vi "FRC Retroreflective Processing Example.vi"(10 "Image Src":T2) -> ()   [LabVIEW 2014]
uses:
  Vision Support Code/Camera Types.ctl
  <vilib>/vision/Image Controls.llb/IMAQ Image.ctl
  <vilib>/vision/NI_Vision_Development_Module.lvlib
panel:
  out "Found Totes":T1(array[cluster])
  in  "Camera Type":T3=enum."MS HD3000 square"
  in  "Aspect Fudge Factor":dbl=1.0
  in  "Score Threshold":dbl=75.0
  in  "Annotate":bool=TRUE
  out "ms to process":u32
  out "Sorted Scores":T4(array[cluster]) {"Aspect Ratio" format="%#_3g"; "Area Score" format="%#_3g"; "X" format="%#_3g"; "Y" format="%#_3g"}
  out "Particles":i32
  in  "Ring Light Color":T5={"Hue"={101.37467765958063, 64.10933859299683}, "Sat"={88.03571428571429, 255.0}, "Val"={133.57142857142858, 255.0}} {"Hue" scale=0.0..255.0 scale format="%#_3g"}
  out "Masked":T2(plugin-control)
  out "Original Image":T2(plugin-control)
  # "Instructions:\nUse Source to select image files from a directory or use a USB or IP camera connected to your laptop.\nUse the Color of a ring light to threshold and build particles. Adjust calibration if needed.\nSmall modifications to the diagram will allow for intensity processing instead of color.\nAnnotations show the rectangle and the scores from top to bottom."
  # "Density Profile"
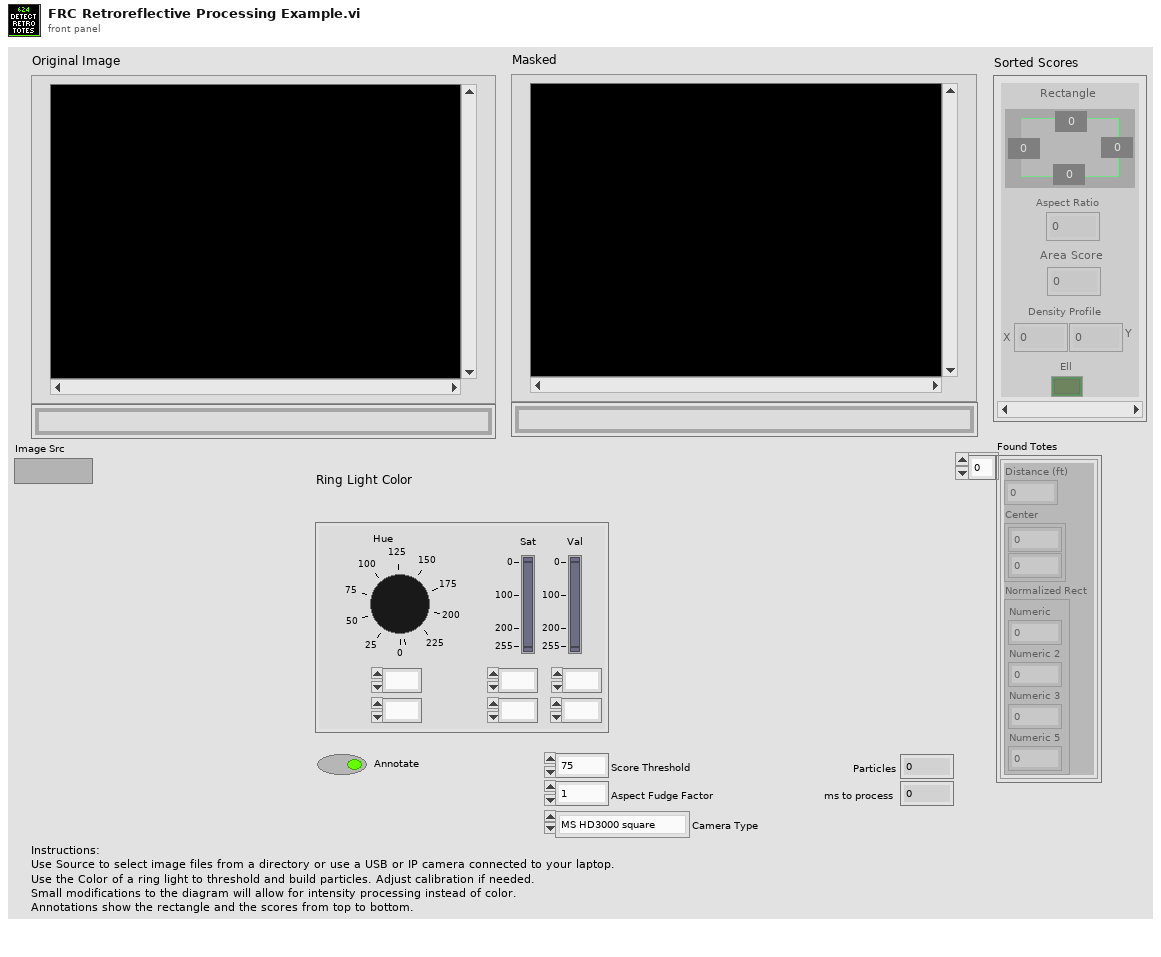
[diagram p1: front panel]
types:
  T1 = cluster{"Distance (ft)":dbl, "Center":cluster{dbl, dbl}, "Normalized Rect":cluster{"Numeric":dbl, "Numeric 2":dbl, "Numeric 3":dbl, "Numeric 5":dbl}}[]
  T2 = typedef "IMAQ Image.ctl" = refnum<image>
  T3 = typedef "Camera Types.ctl" = enum16{"206", "1011", "1013", "MS HD3000 square", "MS HD3000 640x480"}
  T4 = cluster{"Rectangle":cluster{"Numeric":dbl, "Numeric 2":dbl, "Numeric 3":dbl, "Numeric 5":dbl}, "Aspect Ratio":dbl, "Area Score":dbl, "X":dbl, "Y":dbl, "Ell":bool}[]
  T5 = cluster{"Hue":cluster{dbl, dbl}, "Sat":cluster{dbl, dbl}, "Val":cluster{dbl, dbl}}
  T6 = typedef "Particle Parameters" = i32
  T7 = typedef "Image Type" = u32
  T8 = cluster{"Bounding box":cluster{"left":dbl, "top":dbl, "right":dbl, "bottom":dbl}, "Aspect Ratio":dbl, "Area Score":dbl, "X Mask":dbl, "Y Mask":dbl, "Ell":bool}[]
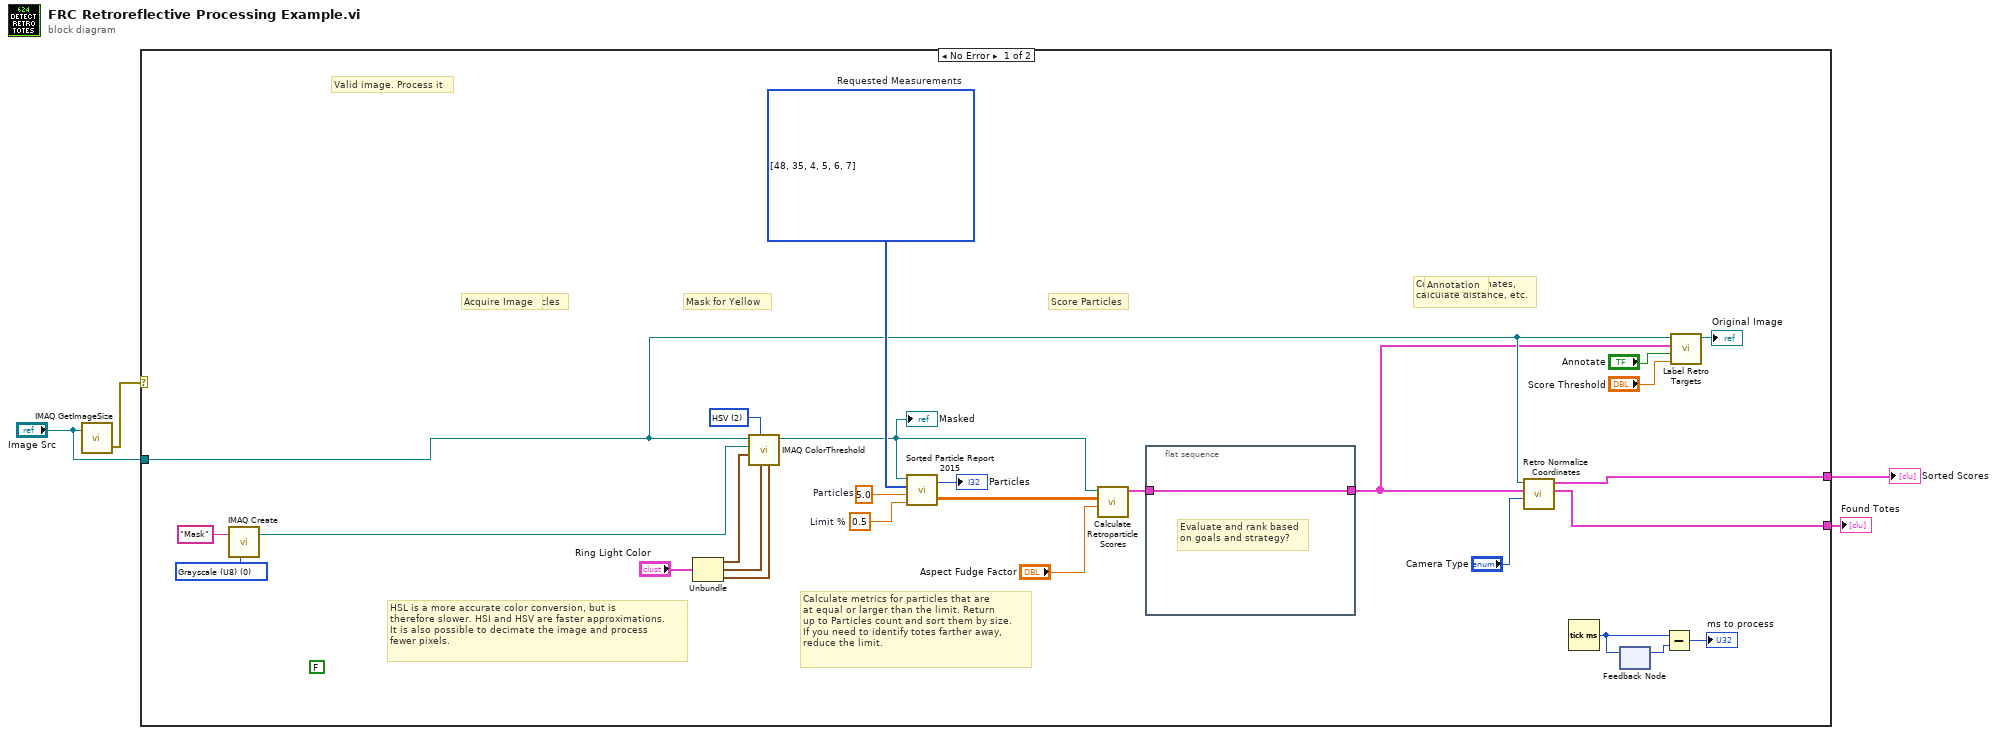
[diagram p0: block diagram]
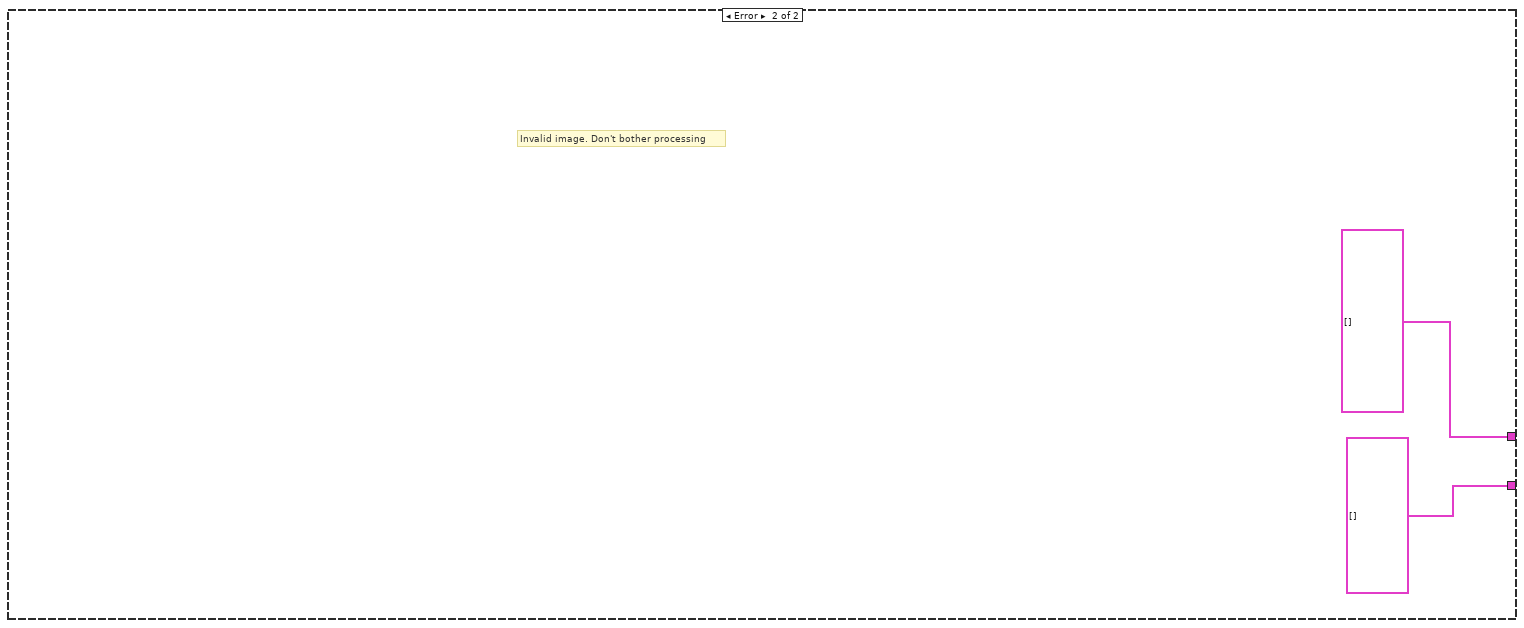
[diagram p2: hidden frame]
diagram:
  n1 = call "IMAQ GetImageSize"("Image"="Image Src") -> ("error out"=w2:errorcluster)  [unwired: 3 in, 2 out]
  n2 = case shown="No Error" w2 {
    tunnel: "Image Src" -> [w27 _]
    tunnel: [w26 T4 [] ("Sorted Scores")] -> w3
    tunnel: [w25 T1 [] ("Found Totes")] -> w1
    frame No Error {
      w17 = 0.5  # Limit %
      w19 = 5.0  # Particles
      w24 = u16 2 items=["RGB", "HSL", "HSV", "HSI"] ("Color Mode")
      (unwired) FALSE
      w28 = T6[] [48, 35, 4, 5, 6, 7] items=["Center of Mass X", "Center of Mass Y", "First Pixel X", "First Pixel Y", "Bounding Rect Left", "Bounding Rect Top", "Bounding Rect Right", "Bounding Rect Bottom", "Max Feret Diameter Start X", "Max Feret Diameter Start Y", "Max Feret Diameter End X", "Max Feret Diameter End Y", "Max Horiz. Segment Length Left", "Max Horiz. Segment Length Right", "Max Horiz. Segment Length Row", "-", "Bounding Rect Width", "Bounding Rect Height", "Bounding Rect Diagonal", "Perimeter", "Convex Hull Perimeter", "Holes' Perimeter", "Max Feret Diameter", "Equivalent Ellipse Major Axis", "Equivalent Ellipse Minor Axis", "Equivalent Ellipse Minor Axis (Feret)", "Equivalent Rect Long Side", "Equivalent Rect Short Side", "Equivalent Rect Diagonal", "Equivalent Rect Short Side (Feret)", "Average Horiz. Segment Length", "Average Vert. Segment Length", "Hydraulic Radius", "Waddel Disk Diameter", "-", "Area", "Holes' Area", "Particle & Holes' Area", "Convex Hull Area", "Image Area", "-", "Number of Holes", "Number of Horiz. Segments", "Number of Vert. Segments", "-", "Orientation", "Max Feret Diameter Orientation", "-", "% Area/Image Area", "% Area/(Particle & Holes' Area)", "Ratio of Equivalent Ellipse Axes", "Ratio of Equivalent Rect Sides", "-", "Elongation Factor", "Compactness Factor", "Heywood Circularity Factor", "Type Factor", "-", "Sum X", "Sum Y", "Sum XX", "Sum XY", "Sum YY", "Sum XXX", "Sum XXY", "Sum XYY", "Sum YYY", "-", "Moment of Inertia XX", "Moment of Inertia XY", "Moment of Inertia YY", "Moment of Inertia XXX", "Moment of Inertia XXY", "Moment of Inertia XYY", "Moment of Inertia YYY", "Norm. Moment of Inertia XX", "Norm. Moment of Inertia XY", "Norm. Moment of Inertia YY", "Norm. Moment of Inertia XXX", "Norm. Moment of Inertia XXY", "Norm. Moment of Inertia XYY", "Norm. Moment of Inertia YYY", "Hu Moment 1", "Hu Moment 2", "Hu Moment 3", "Hu Moment 4", "Hu Moment 5", "Hu Moment 6", "Hu Moment 7"]  # Requested Measurements
      w31 = T7 0 items=["Grayscale (U8)", "Grayscale (I16)", "Grayscale (SGL)", "Complex (CSG)", "RGB (U32)", "HSL (U32)", "RGB (U64)", "Grayscale (U16)"] ("Image Type")
      # "Calculate metrics for particles that are\nat equal or larger than the limit. Return\nup to Particles count and sort them by size.\nIf you need to identify totes farther away,\nreduce the limit."
      # "Measure Particles"
      # "Convert coordinates,\ncalculate distance, etc."
      # "Annotation"
      # "Score Particles"
      # "Mask for Yellow"
      # "Acquire Image"
      # "HSL is a more accurate color conversion, but is\ntherefore slower. HSI and HSV are faster approximations.\nIt is also possible to decimate the image and process\nfewer pixels."
      # "Valid image. Process it"
      n3 = call "IMAQ Create"("Image Name"="Mask", "Image Type"=w31) -> ("New Image"=w29:T2)  [unwired: 2 in, 2 out]
      n4 = Unbundle("Ring Light Color") -> ("Hue"=w23:cluster{dbl, dbl}, "Sat"=w22:cluster{dbl, dbl}, "Val"=w21:cluster{dbl, dbl})
      n5 = call "IMAQ ColorThreshold"("Blue or Luma or Val or Inten Range"=w21, "Green or Sat Range"=w22, "Color Mode"=w24, "Red or Hue Range"=w23, "Image Dst"=w29, "Image Src"=w27) -> ("Image Dst Out"=w13:T2)  [unwired: 4 in, 1 out]
      "Masked" <- w13
      n6 = call "Sorted Particle Report 2015.vi"("Min Area Size %"=w17, "Particle Count Limit"=w19, "Pixel Measurements"=w28, "Image in"=w13) -> ("Sorted Data"=w10:dbl[][], "Particles"=→"Particles":i32)
      n7 = call "Calculate Retroparticle Scores.vi"("Aspect Fudge Factor"="Aspect Fudge Factor", "Sorted Data"=w10, "Image in"=w13) -> ("Scores"=w12:T8)  [unwired: 8 in]
      n8 = flat-sequence {
        tunnel: w12 -> [w32]
        tunnel: [w32] -> w6
        frame #0 {
          # "Evaluate and rank based\non goals and strategy?"
        }
      }
      n9 = call "Retro Normalize Coordinates.vi"("Camera Type"="Camera Type", "Scores"=w6, "Image in"=w27) -> ("Found Totes"=w25:T1, "Sorted Scores"=w26:T4)  [unwired: 7 in]
      n10 = Tick Count (ms)() -> (millisecond timer value=w15:u32)
      n11 = feedback #1() -> (w16:u32)  [unwired: 1 in]
      n12 = feedback-in #1(w15) -> ()
      n13 = Subtract(x=w15, y=w16) -> (x-y=→"ms to process":u32)
      n14 = call "Label Retro Targets.vi"("Score Threshold"="Score Threshold", "Annotate"="Annotate", "Scores"=w6, "Image in"=w27) -> ("Image out"=→"Original Image":T2)  [unwired: 7 in]
    }
    frame Error {
      # "Invalid image. Don't bother processing"
    }
  }
  "Sorted Scores" <- w3
  "Found Totes" <- w1
